vi "MCCMSG Auto Fast Comp.vi"(8 "error in (no error)":errorcluster, 10 "pnError":i32, 11 "hMCCmsg":i32) -> (0 "error out":errorcluster, 2 "pnError out":i32, 3 "function return":i32)   [LabVIEW 2012, in "MultiClamp 700B Controls.lvlib" / "AxMultiClampMsg.lvlib"]
doc: "AXMCCMSG BOOL WINAPI MCCMSG_AutoFastComp(HMCCMSG hMCCmsg, int *pnError);"
uses:
  AxMultiClampMsg.lvlib
  AxMultiClampMsg.dll
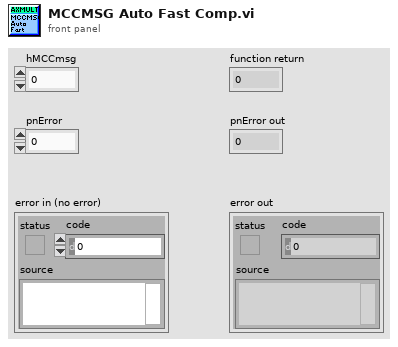
[diagram p1: front panel]
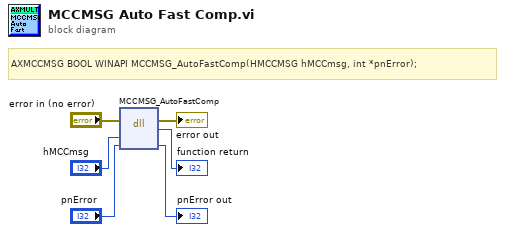
[diagram p0: block diagram]
diagram:
  # "AXMCCMSG BOOL WINAPI MCCMSG_AutoFastComp(HMCCMSG hMCCmsg, int *pnError);"
  n1 = dll-call lib="C:/Users/Southampton/Desktop/Rita/Multiclamp 700B VIs/AxMultiClampMsg/AxMultiClampMsg.*" fn="MCCMSG_AutoFastComp"(error in="error in (no error)", "hMCCmsg"="hMCCmsg", "pnError"="pnError") -> (error out=→"error out":errorcluster, →"function return":i32, "pnError"=→"pnError out":i32)  [unwired: 3 in, 1 out]
